vi "FPControl.vi"(8 "error in":errorcluster, 11 "Function":T1) -> (0 "error out":errorcluster)   [LabVIEW 2014, in "hse-ui.lvlib"]
doc: "____\nHAMPEL SOFTWARE ENGINEERING v0.7.0 (2018-07-16 18:12)"
uses:
  hse-ui.lvlib
  FPControl_Actions.ctl
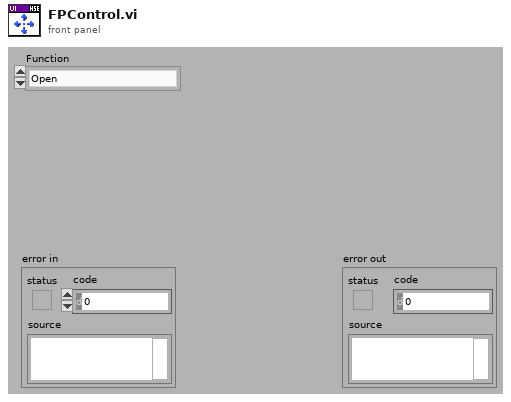
[diagram p1: front panel]
types:
  T1 = typedef "hse-ui.lvlib/FPControl_Actions.ctl" = enum16{"Open", "Hide", "Close", "Bring To Front", "Center", "Minimize", "Maximize"}
  T2 = enum32{"Invalid", "Standard", "Closed", "Hidden", "Minimized", "Maximized"}
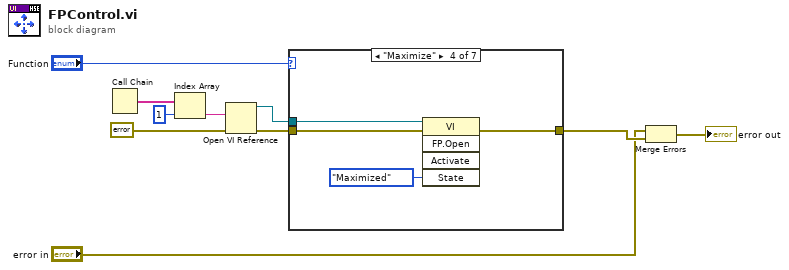
[diagram p0: block diagram]
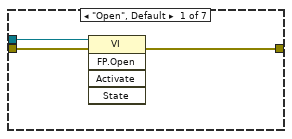
[diagram p2: hidden frame]
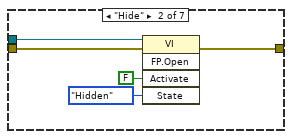
[diagram p3: hidden frame]
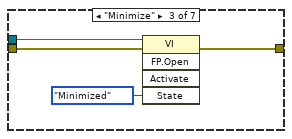
[diagram p4: hidden frame]
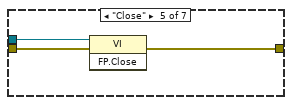
[diagram p5: hidden frame]
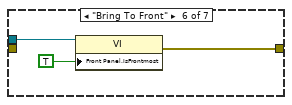
[diagram p6: hidden frame]
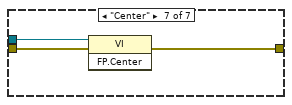
[diagram p7: hidden frame]
diagram:
  n1 = Call Chain() -> (call chain=w7:string[])
  n2 = Index Array(array=w7, index=1) -> (element=w5:string)
  n3 = Open VI Reference(vi path=w5, error in (no error)=errorcluster {"status"=FALSE, "code"=0, "source"=""}) -> (vi reference=w9:refnum<vi>, error out=w10:errorcluster)  [unwired: 1 in, 3 out]
  n4 = case shown="\"Maximize\"" "Function" {
    tunnel: w10 -> [w13 w18 w22 w26 w29 _ w34]
    tunnel: w9 -> [w12 w17 w21 w25 w28 w32 w35]
    tunnel: [w11 w16 w20 w24 w27 w30 w33] -> w3
    frame "Open", Default {
      n5 = invoke class="VI" method="FP.Open"(reference=w12, error in=w13) -> (error out=w11:errorcluster)  [unwired: 3 in, 4 out]
    }
    frame "Hide" {
      n6 = invoke class="VI" method="FP.Open"(reference=w17, error in=w18, "Activate"=FALSE ("Activate?"), "State"=T2."Hidden") -> (error out=w16:errorcluster)  [unwired: 1 in, 4 out]
    }
    frame "Minimize" {
      n7 = invoke class="VI" method="FP.Open"(reference=w21, error in=w22, "State"=T2."Minimized") -> (error out=w20:errorcluster)  [unwired: 2 in, 4 out]
    }
    frame "Maximize" {
      n8 = invoke class="VI" method="FP.Open"(reference=w25, error in=w26, "State"=T2."Maximized") -> (error out=w24:errorcluster)  [unwired: 2 in, 4 out]
    }
    frame "Close" {
      n9 = invoke class="VI" method="FP.Close"(reference=w28, error in=w29) -> (error out=w27:errorcluster)  [unwired: 1 in, 2 out]
    }
    frame "Bring To Front" {
      n10 = property class="VI"(reference=w32, "Front Panel.IsFrontmost"=TRUE) -> (error out=w30:errorcluster)  [unwired: 1 in, 1 out]
    }
    frame "Center" {
      n11 = invoke class="VI" method="FP.Center"(reference=w35, error in=w34) -> (error out=w33:errorcluster)  [unwired: 1 in, 2 out]
    }
  }
  n12 = Merge Errors("error in", w3) -> (→"error out":errorcluster)
